vi "Read tdms file.vi"(8 "error in (no error)":errorcluster, 11 "TDMS-Actor in":refnum<class "TDMS-Actor.lvclass">) -> (0 "error out":errorcluster, 2 "tdms file":refnum<k34>, 3 "TDMS-Actor out":refnum<class "TDMS-Actor.lvclass">)   [LabVIEW 2017, in "BNT_TDMS.lvlib" / "TDMS-Actor.lvclass"]
uses:
  TDMS-Actor.lvclass
  TDMS-Actor.lvclass/TDMS-Actor.ctl
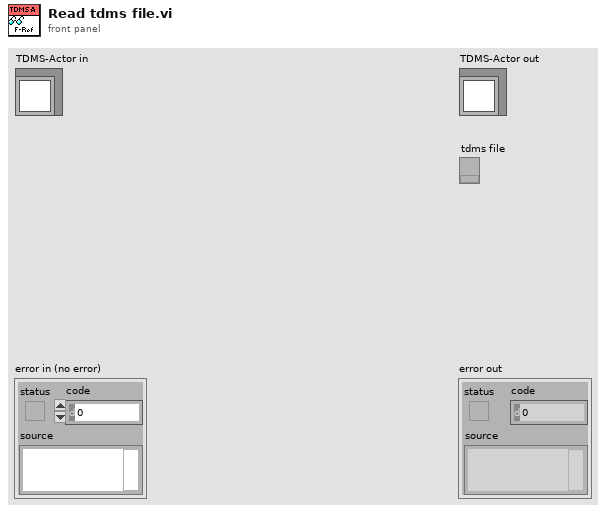
[diagram p1: front panel]
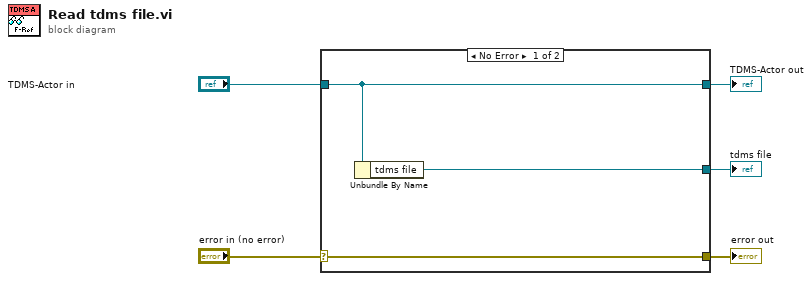
[diagram p0: block diagram]
diagram:
  n1 = case shown="No Error" "error in (no error)" {
    selector: "error in (no error)" -> [w8 w9]
    tunnel: [w8 w9] -> w4
    tunnel: [w7 w10] -> w2
    tunnel: "TDMS-Actor in" -> [w7 w10]
    tunnel: [w6 _] -> w1
    frame No Error {
      n2 = Unbundle By Name(w7) -> ("tdms file"=w6:refnum<k34>)
    }
    frame Error {
    }
  }
  "error out" <- w4
  "TDMS-Actor out" <- w2
  "tdms file" <- w1
